vi "H036 Harsh Pandit SCADA Lab 3b Sem 6.vi"() -> ()   [LabVIEW 2018]
panel:
  in  "Carry In":bool
  in  "Input 2":bool
  in  "Input 1":bool
  out "Carry Out":bool
  out "Sum":bool
  # "Experiment 3b: Develope full adder sub VI using half adder sub VI"
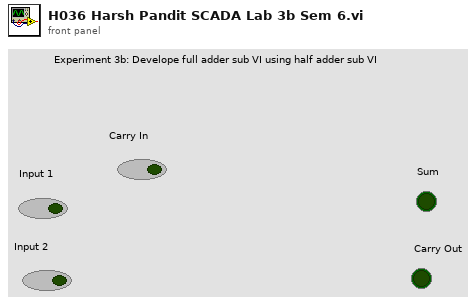
[diagram p1: front panel]
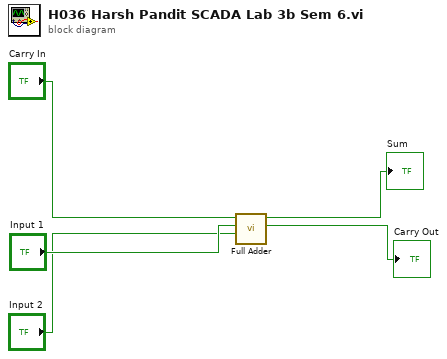
[diagram p0: block diagram]
diagram:
  n1 = call "Full Adder.vi"("Input in"="Input 2", "Input 1"="Input 1", "Carry In"="Carry In") -> ("Carry"=→"Carry Out":bool, "Sum"=→"Sum":bool)  [unwired: 7 in]
